vi "BCD-to-BIN.vi"(1 "Cluster Y":T2) -> (0 "Cluster X":T1)   [LabVIEW 2012]
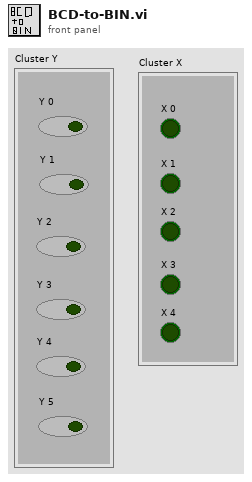
[diagram p1: front panel]
types:
  T1 = cluster{"X 0":bool, "X 1":bool, "X 2":bool, "X 3":bool, "X 4":bool}
  T2 = cluster{"Y 0":bool, "Y 1":bool, "Y 2":bool, "Y 3":bool, "Y 4":bool, "Y 5":bool}
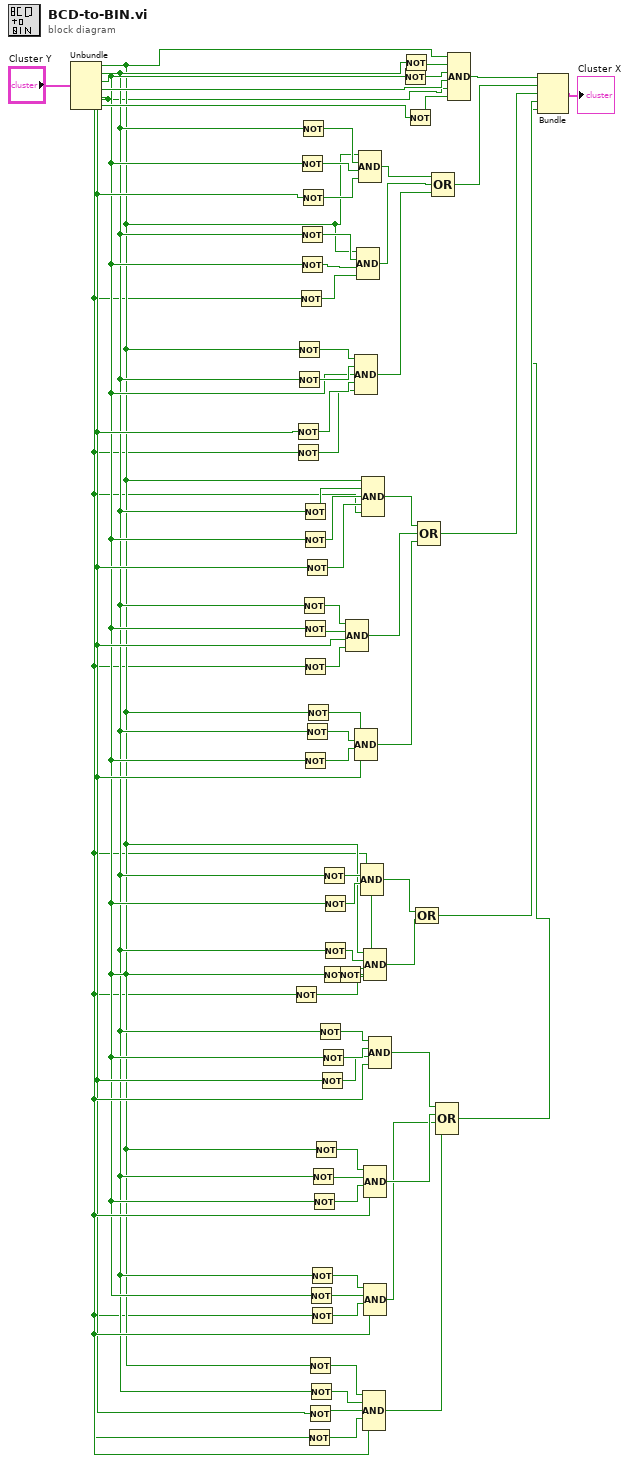
[diagram p0: block diagram]
diagram:
  n1 = Unbundle("Cluster Y") -> ("Y 0"=w3:bool, "Y 1"=w5:bool, "Y 2"=w8:bool, "Y 3"=w9:bool, "Y 4"=w2:bool, "Y 5"=w10:bool)
  n2 = Not(x=w2) -> (.not. x?=w1:bool)
  n3 = Not(x=w9) -> (.not. x?=w49:bool)
  n4 = Not(x=w2) -> (.not. x?=w48:bool)
  n5 = Not(x=w3) -> (.not. x?=w51:bool)
  n6 = Not(x=w5) -> (.not. x?=w50:bool)
  n7 = Not(x=w2) -> (.not. x?=w52:bool)
  n8 = Not(x=w8) -> (.not. x?=w56:bool)
  n9 = Not(x=w5) -> (.not. x?=w54:bool)
  n10 = Not(x=w8) -> (.not. x?=w53:bool)
  n11 = Not(x=w5) -> (.not. x?=w57:bool)
  n12 = Not(x=w9) -> (.not. x?=w55:bool)
  n13 = Not(x=w5) -> (.not. x?=w38:bool)
  n14 = Not(x=w5) -> (.not. x?=w41:bool)
  n15 = Not(x=w8) -> (.not. x?=w42:bool)
  n16 = Not(x=w8) -> (.not. x?=w37:bool)
  n17 = Not(x=w2) -> (.not. x?=w36:bool)
  n18 = Not(x=w8) -> (.not. x?=w39:bool)
  n19 = Not(x=w9) -> (.not. x?=w43:bool)
  n20 = Not(x=w5) -> (.not. x?=w40:bool)
  n21 = Not(x=w3) -> (.not. x?=w7:bool)
  n22 = Not(x=w2) -> (.not. x?=w11:bool)
  n23 = Not(x=w3) -> (.not. x?=w14:bool)
  n24 = Not(x=w9) -> (.not. x?=w12:bool)
  n25 = Not(x=w8) -> (.not. x?=w16:bool)
  n26 = Not(x=w5) -> (.not. x?=w13:bool)
  n27 = Not(x=w5) -> (.not. x?=w17:bool)
  n28 = Not(x=w2) -> (.not. x?=w15:bool)
  n29 = Not(x=w5) -> (.not. x?=w19:bool)
  n30 = Not(x=w8) -> (.not. x?=w18:bool)
  n31 = Not(x=w3) -> (.not. x?=w20:bool)
  n32 = Not(x=w5) -> (.not. x?=w23:bool)
  n33 = Not(x=w9) -> (.not. x?=w21:bool)
  n34 = Not(x=w8) -> (.not. x?=w22:bool)
  n35 = Not(x=w5) -> (.not. x?=w4:bool)
  n36 = Not(x=w8) -> (.not. x?=w31:bool)
  n37 = Not(x=w8) -> (.not. x?=w29:bool)
  n38 = Not(x=w5) -> (.not. x?=w32:bool)
  n39 = Not(x=w3) -> (.not. x?=w30:bool)
  n40 = Compound Arithmetic op=AND(w38, w37, w9, w36) -> (w45:bool)
  n41 = Compound Arithmetic op=AND(w51, w50, w8, w49, w48) -> (w6:bool)
  n42 = Compound Arithmetic op=AND(w7, w40, w39, w9) -> (w44:bool)
  n43 = Compound Arithmetic op=AND(w3, w54, w53, w52) -> (w58:bool)
  n44 = Compound Arithmetic op=AND(w3, w57, w56, w55) -> (w59:bool)
  n45 = Compound Arithmetic op=AND(w30, w4, w29, w2) -> (w34:bool)
  n46 = Compound Arithmetic op=AND(w3, w41, w42, w43, w2) -> (w46:bool)
  n47 = Compound Arithmetic op=AND(w14, w13, w12, w11, w10) -> (w24:bool)
  n48 = Compound Arithmetic op=AND(w3, w32, w31, w1) -> (w33:bool)
  n49 = Compound Arithmetic op=AND(w20, w19, w18, w10) -> (w26:bool)
  n50 = Compound Arithmetic op=AND(w17, w16, w15, w10) -> (w25:bool)
  n51 = Compound Arithmetic op=AND(w23, w22, w21, w10) -> (w27:bool)
  n52 = Not(x=w8) -> (.not. x?=w63:bool)
  n53 = Not(x=w5) -> (.not. x?=w64:bool)
  n54 = Not(x=w10) -> (.not. x?=w62:bool)
  n55 = Compound Arithmetic op=OR(w34, w33) -> (w35:bool)
  n56 = Compound Arithmetic op=OR(w46, w45, w44) -> (w47:bool)
  n57 = Compound Arithmetic op=OR(w59, w58, w6) -> (w60:bool)
  n58 = Compound Arithmetic op=OR(w27, w26, w25, w24) -> (w28:bool)
  n59 = Compound Arithmetic op=AND(w3, w64, w63, w9, w2, w62) -> (w61:bool)
  n60 = Bundle(w61, w60, w47, w35, w28) -> (→"Cluster X":cluster{bool, bool, bool, bool, bool})  [unwired: 1 in]
